vi "relWaypoint.vi"(7 "Base Point":enum16{"Port", "Midpoint", "Starboard"}(ring), 8 "Error In":errorcluster, 9 "Y coord":dbl, 10 "X coord":dbl, 11 "PassBouy.lvclass":refnum<class "PassBouy.lvclass">) -> (0 "Error Out":errorcluster, 1 "Waypoint Out":refnum<class "Waypoint.lvclass">, 3 "PassBouy.lvclass out":refnum<class "PassBouy.lvclass">)   [LabVIEW 2012, in "PassBouy.lvclass"]
doc: "This vi takes in an insance of PassBouy class, the distance the waypoint should be along the line formed by the port and starboard bouy (x-coor), the distance the waypoint should be perpendicular to the line formed by the port and starboard bouy (y-coor). Both the x-coor and the y-coor are relative to the Base point which can be the port bouy, the starboard bouy, and the midpoint they form. If the two bouys are at the exact same location this vi will simply output the location of the bouy."
uses:
  PassBouy.lvclass
  Waypoint/Waypoint.lvclass
  Data/TypeDefs/UTM Location.ctl
  <vilib>/Analysis/Matrix/Datatypes/RealMatrix.ctl
  PassBouy.lvclass/PassBouy.ctl
  <vilib>/Analysis/baseanly.llb/Unit Vector (DBL).vi
  <vilib>/Analysis/Matrix/Numeric/Conversions/Array To Matrix - RA.vi
  <vilib>/Analysis/Matrix/Numeric/Multiply/Multiply - RM,R.vi
  <vilib>/Analysis/Matrix/Numeric/Conversions/Matrix To Array - RM.vi
  <vilib>/Analysis/Matrix/Numeric/Multiply/Multiply - RM,RM.vi
  <vilib>/Analysis/NI_AALBase.lvlib
  <vilib>/Analysis/Matrix/NI_Matrix.lvlib
panel:
  out "output waypoint":T1 {"North" format="%#_10f"; "East" format="%#_8f"}
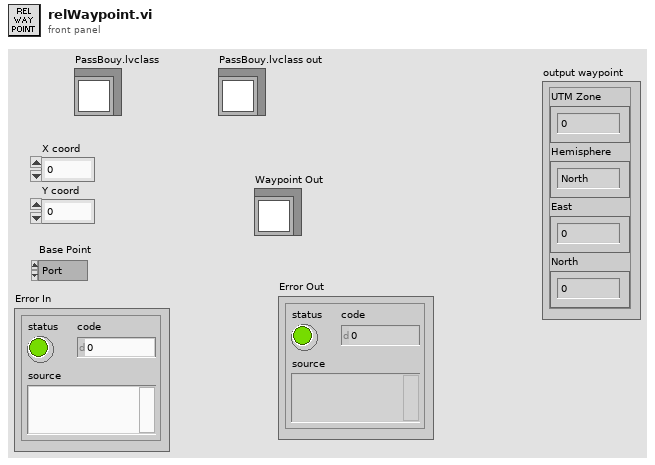
[diagram p1: front panel]
types:
  T1 = typedef "UTM Location.ctl" = cluster{"UTM Zone":dbl, "Hemisphere":enum16{"North", "South"}, "East":dbl, "North":dbl}
  T2 = typedef "NI_Matrix.lvlib/RealMatrix.ctl" = dbl[][]
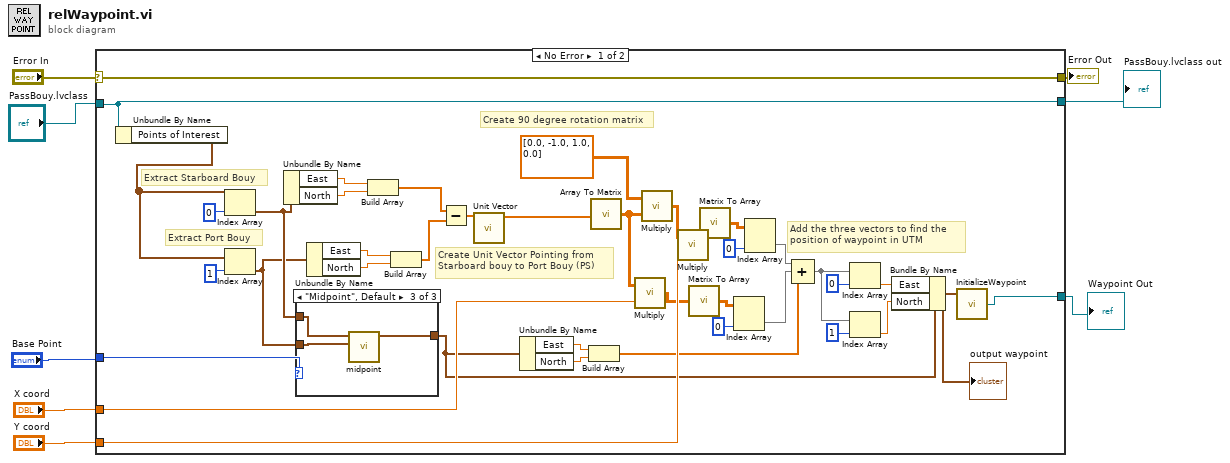
[diagram p0: block diagram]
diagram:
  n1 = case shown="No Error" "Error In" {
    selector: "Error In" -> [w48 w54]
    tunnel: [w48 w54] -> w6
    tunnel: "PassBouy.lvclass" -> [w47 w55]
    tunnel: [w47 w55] -> w7
    tunnel: "X coord" -> [w31 _]
    tunnel: "Y coord" -> [w29 _]
    tunnel: "Base Point" -> [w40 _]
    tunnel: [w16 _] -> w1
    frame No Error {
      # "Add the three vectors to find the \nposition of waypoint in UTM"
      # "Create 90 degree rotation matrix"
      # "Create Unit Vector Pointing from\nStarboard bouy to Port Bouy (PS)"
      # "Extract Port Bouy"
      # "Extract Starboard Bouy"
      n2 = Unbundle By Name(w47) -> ("Points of Interest"=w44:T1[])
      n3 = Index Array(array=w44, index=0) -> (element=w43:T1)
      n4 = Index Array(array=w44, index=1) -> (element=w37:T1)
      n5 = Unbundle By Name(w43) -> ("East"=w42:dbl, "North"=w41:dbl)
      n6 = case shown="\"Midpoint\", Default" w40 {
        tunnel: w43 -> [w49 _ w53]
        tunnel: w37 -> [_ w50 w52]
        tunnel: [w49 w50 w51] -> w15
        frame "Starboard" {
        }
        frame "Port" {
        }
        frame "Midpoint", Default {
          n7 = call "midpoint.vi"("UTM Location 2"=w52, "UTM Location"=w53) -> ("UTM Location 3"=w51:T1)  [unwired: 8 in, 1 out]
        }
      }
      n8 = Unbundle By Name(w37) -> ("East"=w38:dbl, "North"=w39:dbl)
      n9 = Build Array(w42, w41) -> (w36:dbl[])
      n10 = Build Array(w38, w39) -> (w35:dbl[])
      n11 = Subtract(x=w36, y=w35) -> (x-y=w34:dbl[])
      n12 = call-poly <vilib>:"Unit Vector.vi"("Input Vector"=w34) -> ("Unit Vector"=w33:dbl[])  [unwired: 8 in, 2 out]
      n13 = Unbundle By Name(w15) -> ("East"=w28:dbl, "North"=w27:dbl)
      n14 = Build Array(w28, w27) -> (w22:dbl[])
      n15 = call-poly <vilib>:"Array To Matrix.vi"("Real 1D Array"=w33) -> ("Real Matrix (Column Vector)"=w32:T2)
      n16 = call-poly <vilib>:"Multiply.vi"("Real Scalar c"=w31, "Real Matrix A"=w32) -> ("A * c"=w25:T2)
      n17 = call-poly <vilib>:"Multiply.vi"("Real Matrix B"=w32, "Real Matrix A"=T2 [[0.0, -1.0], [1.0, 0.0]] ("matrix")) -> ("A * B"=w30:T2)
      n18 = call-poly <vilib>:"Multiply.vi"("Real Scalar c"=w29, "Real Matrix A"=w30) -> ("A * c"=w17:T2)
      n19 = call-poly <vilib>:"Matrix To Array.vi"("Real Matrix"=w25) -> ("Real 2D Array"=w24:dbl[][])
      n20 = call-poly <vilib>:"Matrix To Array.vi"("Real Matrix"=w17) -> ("Real 2D Array"=w19:dbl[][])
      n21 = Index Array(array=w24, index (col)=0 ("disabled index (col)")) -> (element=w21:dbl[])  [unwired: 1 in]
      n22 = Index Array(array=w19, index (col)=0 ("disabled index (col)")) -> (element=w18:dbl[])  [unwired: 1 in]
      n23 = Compound Arithmetic op=ADD(w18, w21, w22) -> (w10:dbl[])
      n24 = Index Array(array=w10, index=0) -> (element=w12:dbl)
      n25 = Index Array(array=w10, index=1) -> (element=w9:dbl)
      n26 = Bundle By Name(cluster=w15, "East"=w12, "North"=w9) -> (w14:T1)
      "output waypoint" <- w14
      n27 = call "InitializeWaypoint.vi"("Coords"=w14) -> ("Waypoint Out"=w16:refnum<class "Waypoint.lvclass">)  [unwired: 2 in]
    }
    frame Error {
    }
  }
  "Error Out" <- w6
  "PassBouy.lvclass out" <- w7
  "Waypoint Out" <- w1
